vi "parse_get_all_collection_response.vi"(8 "error in (no error)":errorcluster, 10 "body":string, 11 "headers":string) -> (0 "error out":errorcluster, 3 "collection_list":string[](array[string]))   [LabVIEW 2020, in "vector_qdrant.lvclass"]
uses:
  vector_qdrant.lvclass
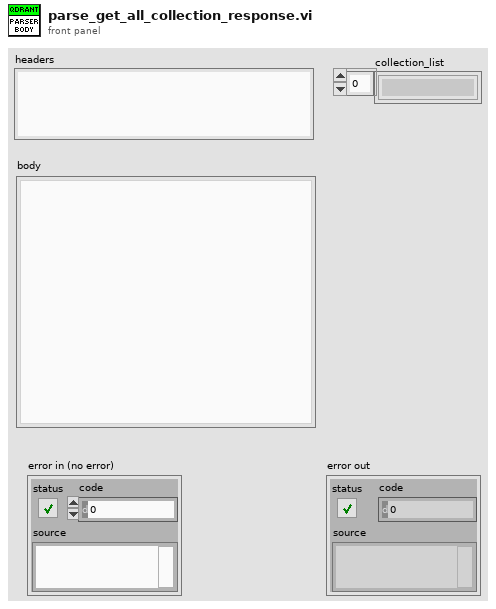
[diagram p1: front panel]
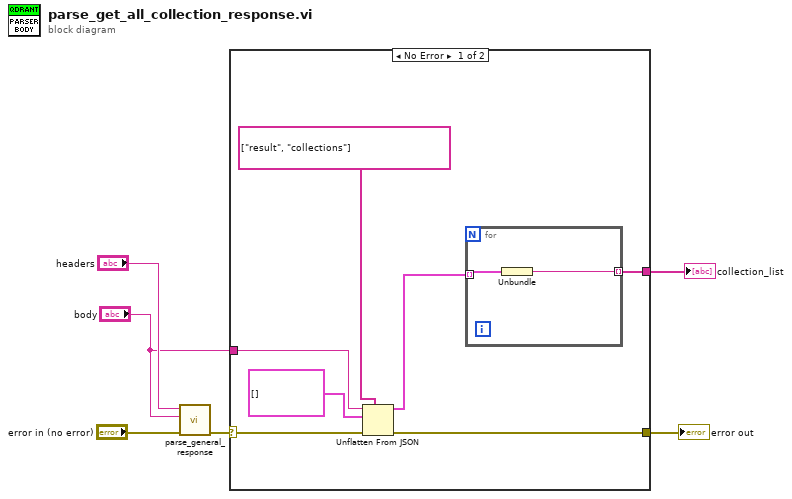
[diagram p0: block diagram]
diagram:
  n1 = call "parse_general_response.vi"("error in (no error)"="error in (no error)", "body"="body", "headers"="headers") -> ("error out"=w3:errorcluster)  [unwired: 8 in]
  n2 = case shown="No Error" w3 {
    selector: w3 -> [w13 w16]
    tunnel: [w7 w16] -> w6
    tunnel: "body" -> [w11 _]
    tunnel: [w8 _] -> w5
    frame No Error {
      n3 = Unflatten From JSON(path=string[] ["result", "collections"], JSON string=w11, type and defaults=cluster{"name":string}[] [], error in (no error)=w13) -> (value=w9:cluster{"name":string}[], error out=w7:errorcluster)  [unwired: 3 in]
      n4 = for {
        tunnel: w9 -> [w15] mode=indexing
        tunnel: [w14] -> w8 mode=indexing
        n5 = Unbundle(w15) -> ("name"=w14:string)
      }
    }
    frame Error {
    }
  }
  "error out" <- w6
  "collection_list" <- w5
